vi "Write GaugeController Obj.vi"(8 "error in (no error)":errorcluster, 10 "GaugeController.lvclass":refnum<class "GaugeController.lvclass">, 11 "GaugeController Configuration in":refnum<class "GaugeController Configuration.lvclass">) -> (0 "error out":errorcluster, 3 "GaugeController Configuration out":refnum<class "GaugeController Configuration.lvclass">)   [LabVIEW 2016, in "Hardware.lvlib" / "GaugeController.lvlib" / "GaugeController Configuration.lvclass"]
uses:
  <userlib>/Common Components/Hardware/GaugeController/GaugeController Config/GaugeController Configuration.lvclass
  <userlib>/Common Components/Hardware/GaugeController/GaugeController/GaugeController.lvclass
  <userlib>/Common Components/Hardware/GaugeController/GaugeController Config/GaugeController Configuration.lvclass/GaugeController Configuration.ctl
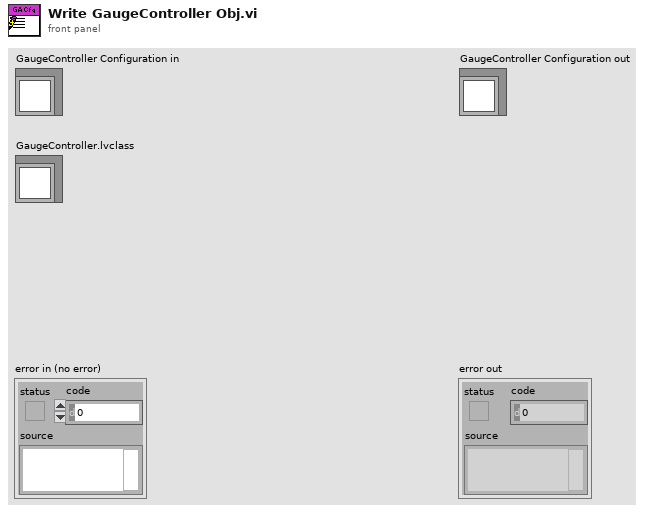
[diagram p1: front panel]
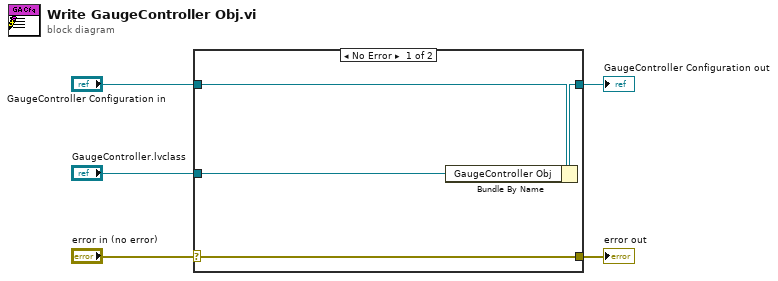
[diagram p0: block diagram]
diagram:
  n1 = case shown="No Error" "error in (no error)" {
    selector: "error in (no error)" -> [w9 w10]
    tunnel: [w9 w10] -> w4
    tunnel: [w7 w11] -> w2
    tunnel: "GaugeController Configuration in" -> [w8 w11]
    tunnel: "GaugeController.lvclass" -> [w6 _]
    frame No Error {
      n2 = Bundle By Name(cluster=w8, "GaugeController Obj"=w6) -> (w7:refnum<class "GaugeController Configuration.lvclass">)
    }
    frame Error {
    }
  }
  "error out" <- w4
  "GaugeController Configuration out" <- w2
